vi "MRayBallTracking.vi"(11 "CameraDevRef":T1) -> ()   [LabVIEW 2011]
uses:
  <vilib>/Rock Robotics/WPI/Camera/WPI_CameraDevRef.ctl
  Robot Global Data.vi
  <vilib>/vision/NI_Vision_Development_Module.lvlib
panel:
  in  "error in (no error)":errorcluster
  in  "View 2":bool
  in  "Processing":enum32{"Color", "Intensity", "Intensity Open"}(tab)=enum."Intensity"
  in  "Luminance":i32=255
  in  "Saturation":i32=255
  in  "Hue":i32(knob)=65 scale=0.0..255.0
  in  "Margins":cluster{"Hue":i32, "Sat":i32, "Lum":i32}={"Hue"=20, "Sat"=27, "Lum"=30} {"Sat" scale=0.0..40.0; "Lum" scale=0.0..40.0; "Hue" scale=0.0..40.0}
  in  "Range":cluster{"Lower value":sgl, "Upper value":sgl}={"Lower value"=107.17391, "Upper value"=255.0} {"Lower value" scale=0.0..255.0; "Upper value" scale=0.0..255.0}
  in  "Range 2":cluster{"Lower value":sgl, "Upper value":sgl}={"Lower value"=123.804344, "Upper value"=255.0} {"Lower value" scale=0.0..255.0; "Upper value" scale=0.0..255.0}
  in  "Particle Count Limit":i32=8
  in  "Area Size Limit":i32=444
  in  "Score Limits":T2={"Rect Coverage"=76.0, "Aspect Ratio"=40.0, "X Edge Strength"=40.0, "Y Edge Strength"=60.0}
  out "Target Info":T3(array[cluster])
  in  "View":bool
  out "Original Image":T4(plugin-control)
  out "Processed Image":T4(plugin-control)
  out "Aspect Ratio":dbl[](array[numeric])
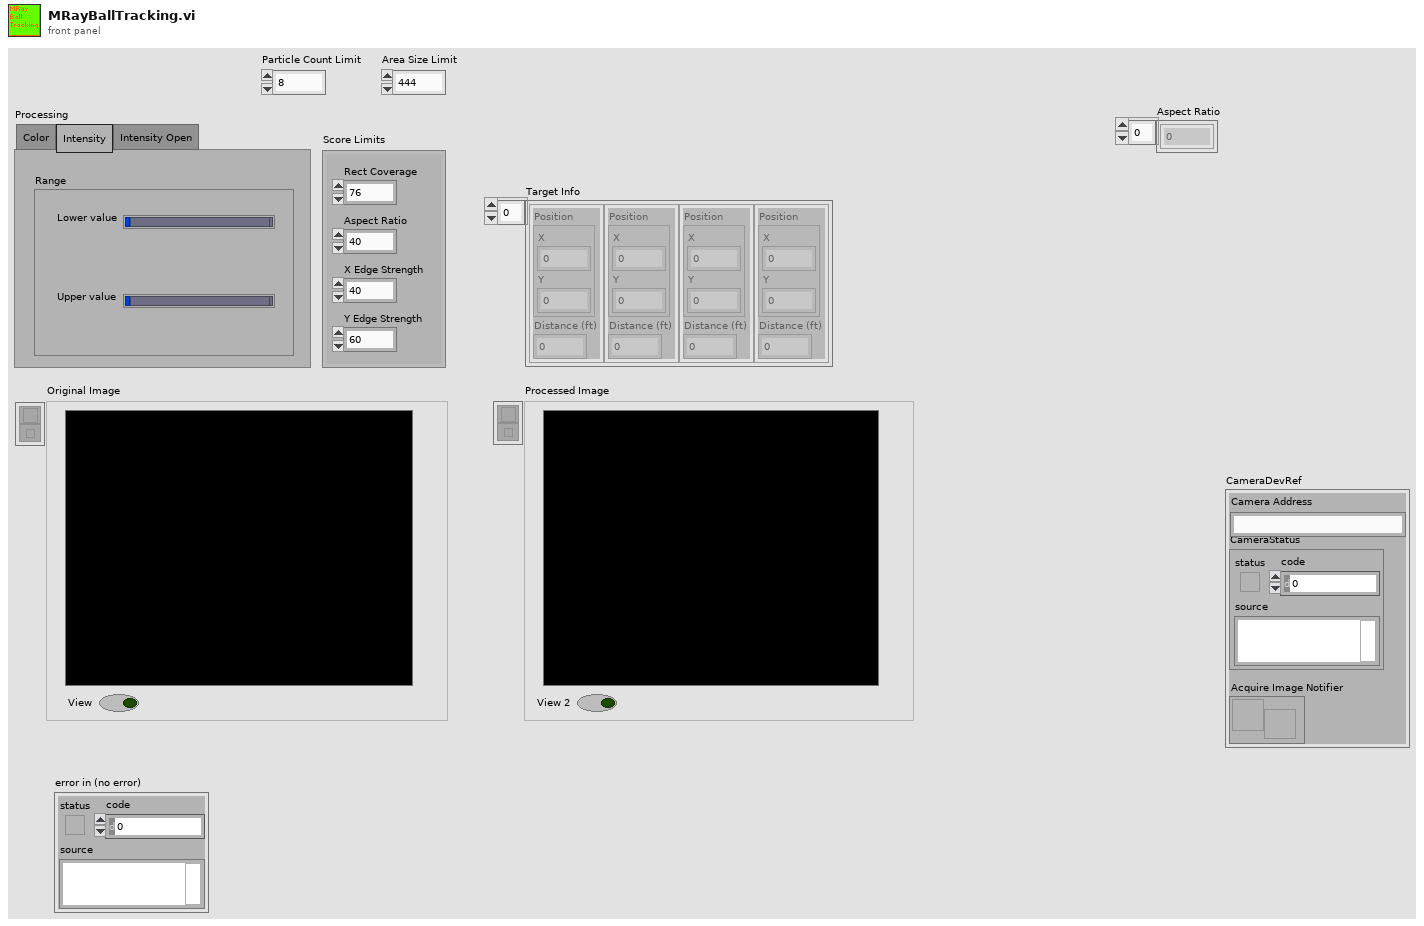
[diagram p1: front panel]
types:
  T1 = typedef "WPI_CameraDevRef.ctl" = cluster{"Camera Address":string, "CameraStatus":errorcluster, "Acquire Image Notifier":refnum<notifier>}
  T2 = cluster{"Rect Coverage":dbl, "Aspect Ratio":dbl, "X Edge Strength":dbl, "Y Edge Strength":dbl}
  T3 = cluster{"Position":cluster{"X":dbl, "Y":dbl}, "Distance (ft)":dbl}[]
  T4 = typedef "IMAQ Image.ctl" = refnum<image>
  T5 = typedef "Image Type" = u32
  T6 = enum32{"AutoM", "Close", "Dilate", "Erode", "Gradient", "Gradient out", "Gradient in", "Hit miss", "Open", "PClose", "POpen", "Thick", "Thin"}
  T7 = typedef "WPI_CameraImageSize.ctl" = enum16{"640x480", "320x240", "160x120"}
  T8 = cluster{"fps":i32, "compression":i32, "Image Size":T7}
  T9 = cluster{cluster{"Left":dbl, "Top":dbl, "Right":dbl, "Bottom":dbl}, dbl[]}[]
  T10 = cluster{"Left":dbl, "Top":dbl, "Right":dbl, "Bottom":dbl}
  T11 = cluster{"Target Center (-1 to 1)":cluster{"X":dbl, "Y":dbl}, "Distance (ft)":dbl}
  T12 = cluster{"Target Center (-1 to 1)":cluster{"X":dbl, "Y":dbl}, "Distance (ft)":dbl}[]
  T13 = cluster{"Score Limits[0]":dbl, "Score Limits[1]":dbl, "Score Limits[2]":dbl, "Score Limits[3]":dbl, "Score Limits[4]":dbl, "Score Limits[5]":dbl, "Score Limits[6]":dbl, "Score Limits[7]":dbl, "Score Limits[8]":dbl}
  T14 = cluster{"Score Limits[0]":dbl, "Score Limits[1]":dbl}
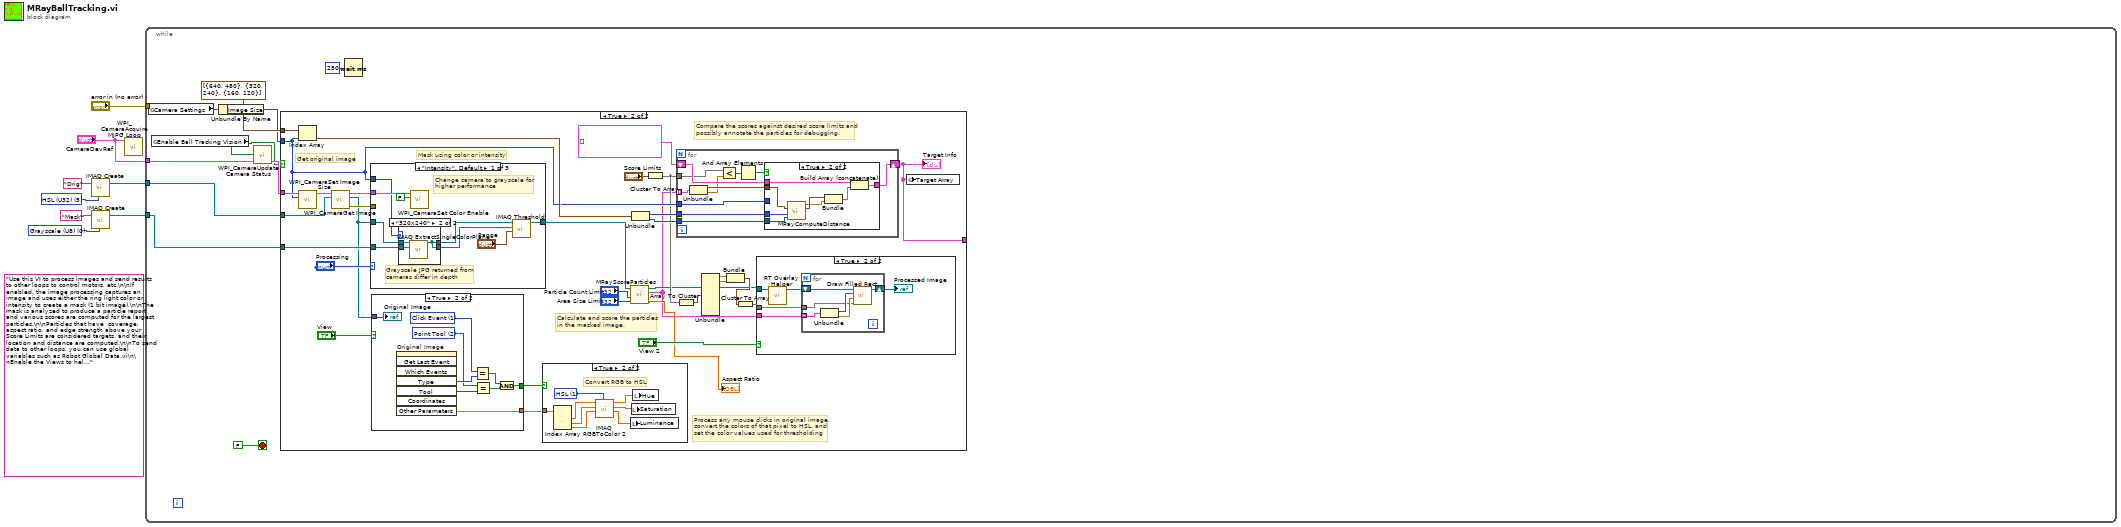
[diagram p0: block diagram]
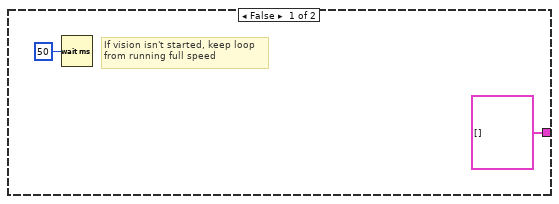
[diagram p2: hidden frame]
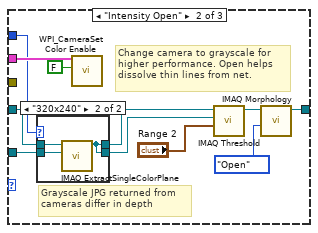
[diagram p5: hidden frame]
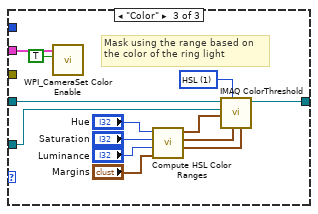
[diagram p7: hidden frame]
diagram:
  w3 = T5 0 items=["Grayscale (U8)", "Grayscale (I16)", "Grayscale (SGL)", "Complex (CSG)", "RGB (U32)", "HSL (U32)", "RGB (U64)", "Grayscale (U16)"] ("Image Type")
  (unwired) "Use this VI to process images and send results to other loops to control motors, etc.\n\nIf enabled, the image processing captures an image and uses either the ring light color or intensity to create a mask (1 bit image).\n\nThe mask is analyzed to produce a particle report and various scores are computed for the largest particles.\n\nParticles that have  coverage, aspect ratio, and edge strength above your Score Limits are considered targets, and their location and distance are computed.\n\nTo send data to other loops, you can use global variables such as Robot Global Data.vi\n\nEnable the Views to help debug color settings. Disable the View to speed up processing."
  w7 = T5 5 items=["Grayscale (U8)", "Grayscale (I16)", "Grayscale (SGL)", "Complex (CSG)", "RGB (U32)", "HSL (U32)", "RGB (U64)", "Grayscale (U16)"] ("Image Type")
  n1 = call "IMAQ Create"("Image Name"="Orig", "Image Type"=w7) -> ("New Image"=w6:T4)  [unwired: 2 in, 2 out]
  n2 = call "IMAQ Create"("Image Name"="Mask", "Image Type"=w3) -> ("New Image"=w1:T4)  [unwired: 2 in, 2 out]
  n3 = call <vilib>:"WPI_CameraAcquire MJPG Loop.vi"("CameraDevRef"="CameraDevRef") -> ()  [unwired: 11 in]
  n4 = while {
    tunnel: w6 -> [w17]
    tunnel: "CameraDevRef" -> [w16]
    tunnel: "error in (no error)" -> [_]
    tunnel: w1 -> [w13]
    stop <- FALSE stop-if-true
    n5 = global read "Robot Global Data.vi" "Camera Settings"() -> (w11:T8)
    n6 = global read "Robot Global Data.vi" "Enable Ball Tracking Vision"() -> (w14:bool)
    n7 = Unbundle By Name(w11) -> ("Image Size"=w10:T7)
    n8 = call <vilib>:"WPI_CameraUpdate Camera Status.vi"("CameraDevRef In"=w16, "Enable Vision"=w14) -> ("CameraDevRef Out"=w15:T1)  [unwired: 3 in]
    n9 = case shown="True" w14 {
      tunnel: w17 -> [_ w48]
      tunnel: w15 -> [_ w44]
      tunnel: w13 -> [_ w36]
      tunnel: cluster{i32, i32}[] [{640, 480}, {320, 240}, {160, 120}] -> [_ w40]
      tunnel: w10 -> [_ w33]
      tunnel: [T3 [] w34] -> _
      frame False {
        # "If vision isn't started, keep loop\nfrom running full speed"
        n10 = Wait (ms)(milliseconds to wait=u32 50) -> ()  [unwired: 1 out]
      }
      frame True {
        # "Compare the scores against desired score limits and\npossibly annotate the particles for debugging."
        # "Process any mouse clicks in original image,\nconvert the colors of that pixel to HSL, and\nset the color values used for thresholding"
        # "Calculate and score the particles\nin the masked image."
        # "Mask using color or intensity"
        # "Get original image"
        n11 = call <vilib>:"WPI_CameraSet Image Size.vi"("Image Size"=w33, "CameraDevRef"=w44) -> ("CameraDevRef Out"=w45:T1)  [unwired: 8 in, 1 out]
        n12 = Index Array(array=w40, index=w33) -> (element=w37:cluster{i32, i32})
        n13 = call <vilib>:"WPI_CameraGet Image.vi"("Image"=w48, "CameraDevRef"=w45) -> ("error out"=w46:errorcluster, "Image Out"=w35:T4, "CameraDevRef Out"=w47:T1)  [unwired: 7 in]
        n14 = case shown="\"Intensity\", Default" "Processing" {
          tunnel: w35 -> [w65 w77 w103]
          tunnel: [w68 w82 w102] -> w26
          tunnel: w47 -> [w66 w80 w93]
          tunnel: w46 -> [_ _ _]
          tunnel: w36 -> [w64 w78 w91]
          tunnel: w33 -> [w63 w79 _]
          frame "Intensity", Default {
            # "Grayscale JPG returned from\ncameras differ in depth"
            # "Change camera to grayscale for\nhigher performance"
            n15 = case shown="\"320x240\"" w63 {
              tunnel: w65 -> [w71 w74]
              tunnel: w64 -> [w70 w73]
              tunnel: [w71 w72] -> w62
              tunnel: [w70 w72] -> w61
              frame "640x480", Default {
              }
              frame "320x240" {
                n16 = call "IMAQ ExtractSingleColorPlane"("Image Dst"=w73, "Image Src"=w74) -> ("Image Dst Out"=w72:T4)  [unwired: 8 in, 1 out]
              }
            }
            n17 = call <vilib>:"WPI_CameraSet Color Enable.vi"("Color Enabled"=FALSE, "CameraDevRef"=w66) -> ()  [unwired: 8 in, 2 out]
            n18 = call "IMAQ Threshold"("Range"="Range", "Image Dst"=w61, "Image Src"=w62) -> ("Image Dst Out"=w68:T4)  [unwired: 3 in, 5 out]
          }
          frame "Intensity Open" {
            # "Grayscale JPG returned from\ncameras differ in depth"
            # "Change camera to grayscale for\nhigher performance. Open helps\ndissolve thin lines from net."
            n19 = case shown="\"320x240\"" w79 {
              tunnel: w77 -> [w87 w90]
              tunnel: w78 -> [w86 w89]
              tunnel: [w87 w88] -> w76
              tunnel: [w86 w88] -> w75
              frame "640x480", Default {
              }
              frame "320x240" {
                n20 = call "IMAQ ExtractSingleColorPlane"("Image Dst"=w89, "Image Src"=w90) -> ("Image Dst Out"=w88:T4)  [unwired: 8 in, 1 out]
              }
            }
            n21 = call <vilib>:"WPI_CameraSet Color Enable.vi"("Color Enabled"=FALSE, "CameraDevRef"=w80) -> ()  [unwired: 8 in, 2 out]
            n22 = call "IMAQ Threshold"("Range"="Range 2", "Image Dst"=w75, "Image Src"=w76) -> ("Image Dst Out"=w83:T4)  [unwired: 3 in, 5 out]
            n23 = call "IMAQ Morphology"("Operation"=T6."Open", "Image Src"=w83) -> ("Image Dst Out"=w82:T4)  [unwired: 8 in, 1 out]
          }
          frame "Color" {
            w101 = u16 1 items=["RGB", "HSL", "HSV", "HSI"] ("Color Mode")
            # "Mask using the range based on\nthe color of the ring light"
            n24 = call <vilib>:"WPI_CameraSet Color Enable.vi"("Color Enabled"=TRUE, "CameraDevRef"=w93) -> ()  [unwired: 8 in, 2 out]
            n25 = call "Compute HSL Color Ranges.vi"("Margins"="Margins", "Luminance"="Luminance", "Saturation"="Saturation", "Hue"="Hue") -> ("Lum Range"=w98:cluster{i32, i32}, "Sat Range"=w99:cluster{i32, i32}, "Hue Range"=w100:cluster{i32, i32})  [unwired: 5 in]
            n26 = call "IMAQ ColorThreshold"("Blue or Luma or Val or Inten Range"=w98, "Green or Sat Range"=w99, "Color Mode"=w101, "Red or Hue Range"=w100, "Image Dst"=w91, "Image Src"=w103) -> ("Image Dst Out"=w102:T4)  [unwired: 4 in, 1 out]
          }
        }
        n27 = case shown="True" "View" {
          tunnel: w35 -> [_ w123]
          tunnel: [_ w118] -> w42
          tunnel: [_ w115] -> w41
          frame False {
          }
          frame True {
            w116 = 2 items=["None", "Selection Tool", "Point Tool", "Line Tool", "Rectangle Tool", "Oval Tool", "Polygon Tool", "ClosedFreehandTool", "Annulus Tool", "Rotated Rectangle Tool", "Zoom Tool", "Pan Tool", "Polyline Tool", "Freehand Tool"] ("Tool")
            w117 = 1 items=["No Event"=0, "Click Event"=1, "Draw Event"=2, "Size Event"=4, "Scroll Event"=5, "Double Click Event"=8] ("Type")
            n28 = invoke on="Original Image" class="ImageControl" method="Get Last Event"() -> ("Type"=w119:i32, "Tool"=w122:i32, "Other Parameters"=w115:sgl[])  [unwired: 8 in, 5 out]
            n29 = Equal?(x=w117, y=w119) -> (x = y?=w120:bool)
            n30 = Equal?(x=w116, y=w122) -> (x = y?=w121:bool)
            n31 = And(x=w120, y=w121) -> (x .and. y?=w118:bool)
            "Original Image" <- w123
          }
        }
        n32 = case shown="True" w42 {
          tunnel: w41 -> [_ w60]
          frame False {
          }
          frame True {
            w59 = u16 1 items=["RGB", "HSL", "HSV", "HSI", "CIE L*a*b*", "CIE XYZ"] ("Color Mode")
            # "Convert RGB to HSL"
            n33 = Index Array(array=w60) -> (element #1=w58:sgl, element #2=w56:sgl, element #3=w54:sgl)  [unwired: 3 in]
            n34 = call "IMAQ RGBToColor 2"("Color Mode"=w59, "Blue value"=w54, "Green value"=w56, "Red value"=w58) -> ("Blue or Luma or Val or Inten or Z or b*value"=w53:dbl, "Green or Sat or Y or a* value"=w55:dbl, "Red or Hue or X or L* value"=w57:dbl)  [unwired: 4 in, 1 out]
            n35 = local write "Luminance"(w53) -> ()
            n36 = local write "Saturation"(w55) -> ()
            n37 = local write "Hue"(w57) -> ()
          }
        }
        n38 = call "MRayScoreParticles.vi"("Area Size Limit"="Area Size Limit", "Particle Count Limit"="Particle Count Limit", "Image Refnum in"=w26) -> ("Aspect Ratio"=→"Aspect Ratio":dbl[], "Scored Particle Info"=w21:T9, "Image Refnum out"=w23:T4)  [unwired: 6 in]
        n39 = Unbundle(w37) -> (w39:i32, w38:i32)
        n40 = Cluster To Array(cluster="Score Limits") -> (array=w32:dbl[])
        n41 = for {
          shift-right: [w133] -> w34
          shift-left: T3 [] -> [w134]
          tunnel: w39 -> [w132]
          tunnel: w21 -> [w130] mode=indexing
          tunnel: w32 -> [w125]
          tunnel: w33 -> [w129]
          tunnel: w38 -> [w124]
          n42 = Unbundle(w130) -> (w131:T10, w126:dbl[])
          n43 = Less?(x=w125, y=w126) -> (x < y?=w128:bool[])
          n44 = And Array Elements(Boolean array=w128) -> (logical AND=w127:bool)
          n45 = case shown="True" w127 {
            tunnel: w134 -> [w135 w143]
            tunnel: [w135 w142] -> w133
            tunnel: w131 -> [_ w141]
            tunnel: w132 -> [_ w140]
            tunnel: w129 -> [_ _]
            tunnel: w124 -> [_ w139]
            frame False {
            }
            frame True {
              n46 = call "MRayComputeDistance.vi"("Y Image Resolution"=w139, "X Image Resolution"=w140, "Bounding Box"=w141) -> ("Target Center (-1 to 1)"=w137:cluster{"X":dbl, "Y":dbl}, "Distance (ft)"=w136:dbl)  [unwired: 7 in]
              n47 = Bundle("Target Center (-1 to 1)"=w137, "Distance (ft)"=w136) -> (w138:T11)  [unwired: 1 in]
              n48 = Build Array (concatenate)(w143, w138) -> (w142:T12)
            }
          }
        }
        "Target Info" <- w34
        n49 = Array To Cluster(array=w32) -> (cluster=w31:T13)
        n50 = Unbundle(w31) -> ("Score Limits[0]"=w30:dbl, "Score Limits[1]"=w29:dbl)  [unwired: 7 out]
        n51 = Bundle("Score Limits[0]"=w30, "Score Limits[1]"=w29) -> (w28:T14)  [unwired: 1 in]
        n52 = Cluster To Array(cluster=w28) -> (array=w27:dbl[])
        n53 = case shown="True" "View 2" {
          tunnel: w23 -> [_ w105]
          tunnel: w21 -> [_ w107]
          tunnel: w27 -> [_ w106]
          frame False {
          }
          frame True {
            n54 = call "RT Overlay Helper.vi"("Refnum in"=w105) -> ("Refnum out"=w108:T4)  [unwired: 10 in]
            n55 = for {
              shift-right: [w113] -> w104
              shift-left: w108 -> [w114]
              tunnel: w107 -> [w110] mode=indexing
              tunnel: w106 -> [w109]
              n56 = Unbundle(w110) -> (w111:T10, w112:dbl[])
              n57 = call "Draw Filled Rect.vi"("Limits"=w109, "Scores"=w112, "Bounding Box"=w111, "image in"=w114) -> ("image out"=w113:T4)  [unwired: 7 in]
            }
            "Processed Image" <- w104
          }
        }
        n58 = global write "Robot Global Data.vi" "Target Array"(w34) -> ()
      }
    }
    n59 = Wait (ms)(milliseconds to wait=u32 250) -> ()  [unwired: 1 out]
  }
